vi "Actor Core.vi"(8 "error in":errorcluster, 11 "Nested in":refnum<class "UI_CAFÉ_MEX_ESP.lvclass">) -> (0 "error out":errorcluster, 3 "Actor out":refnum<class "Actor.lvclass">)   [LabVIEW 2019, in "DATA_UI_CAFÉ_MEX_ESP.lvlib" / "UI_CAFÉ_MEX_ESP.lvclass"]
doc: "(<B>Filename</B>: Actor Framework.lvlib:Actor.lvclass:Actor Core.vi)\n\nReceives messages to the actor, reacts to them, and initiates any error handling that may shut the actor down.\n\nDescendant classes may override this VI to append parallel tasks for the actor to complete while it handles messages. Overrides use the Call Parent Method node."
uses:
  C:/Program Files (x86)/National Instruments/LabVIEW 2019/vi.lib/ActorFramework/Actor/Actor.lvclass
  <vilib>/ActorFramework/Actor/Actor.lvclass
  <vilib>/ActorFramework/Actor/Actor.lvclass/Actor.ctl
  <vilib>/ActorFramework/Message Enqueuer/Message Enqueuer.lvclass/Message Enqueuer.ctl
  Write VI Refnum.vi
  <vilib>/ActorFramework/Message Enqueuer/Init from Existing Queue.vi
  <vilib>/ActorFramework/Message Enqueuer/Enqueue.vi
  <vilib>/ActorFramework/Stop Msg/Stop Msg.lvclass
  C:/Program Files (x86)/National Instruments/LabVIEW 2019/vi.lib/ActorFramework/Message/Message.lvclass
  <vilib>/ActorFramework/Message Priority Queue/Priority Enqueue.vi
  <vilib>/ActorFramework/Message Enqueuer/Message Enqueuer.lvclass
panel:
  in  "COMPRAR MERCANCÍA":bool
  in  "10 PESOS MEXICANOS":bool
  in  "5 PESOS MEXICANOS":bool
  in  "2 PESOS MEXICANOS":bool
  in  "1 PESO MEXICANO":bool
  out "CRÉDITO":dbl
  out "MONEDA":string
  out "PRODUCTO":string
  out "CANTIDAD":dbl
  out "PRECIO":dbl
  in  "SOLICITAR MERCANCIA":bool
  in  "MERCANCÍA":i32(listbox)
  # "INFORMACIÓN DEL PRODUCTO SELECCIONADO"
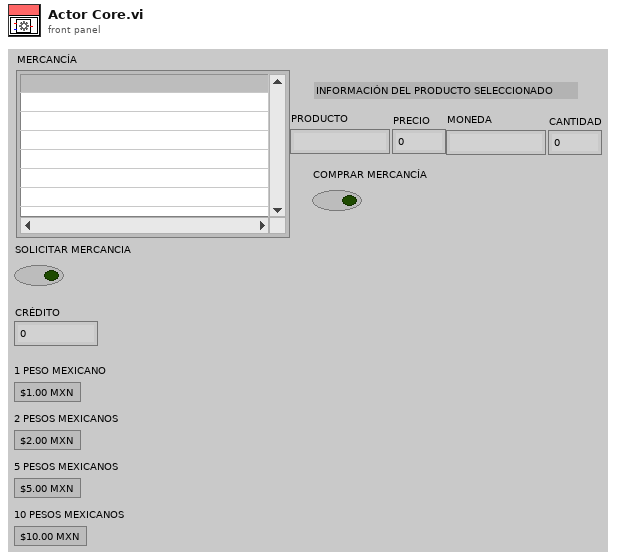
[diagram p1: front panel]
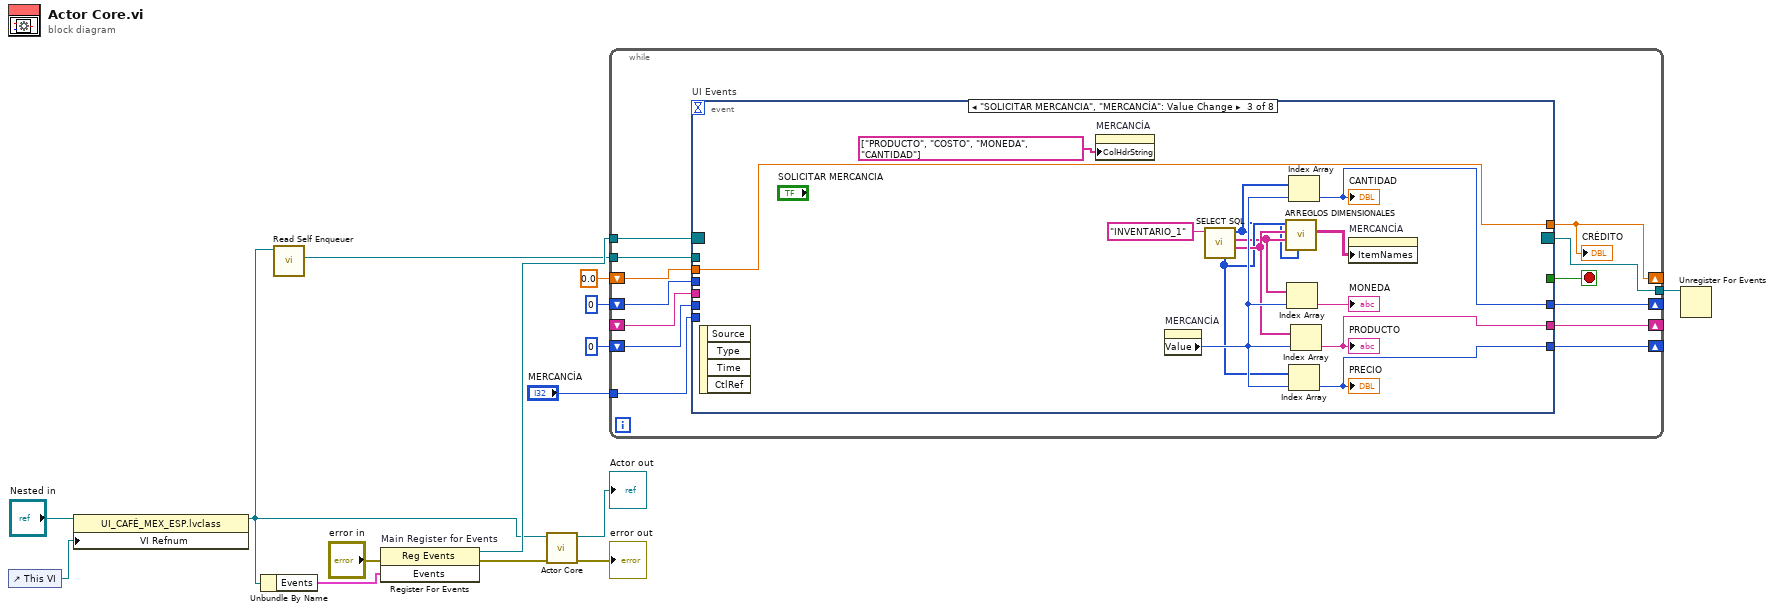
[diagram p0: block diagram]
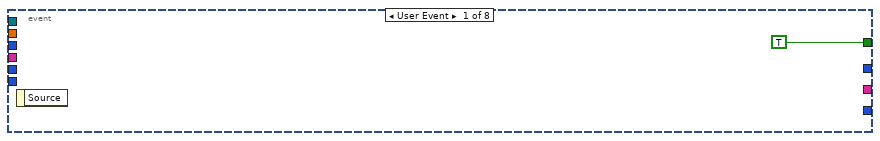
[diagram p2: hidden frame]
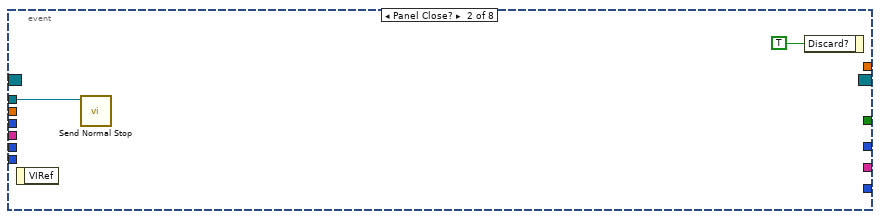
[diagram p3: hidden frame]
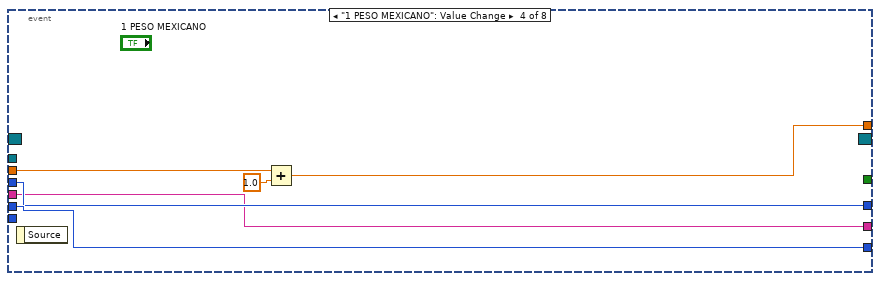
[diagram p4: hidden frame]
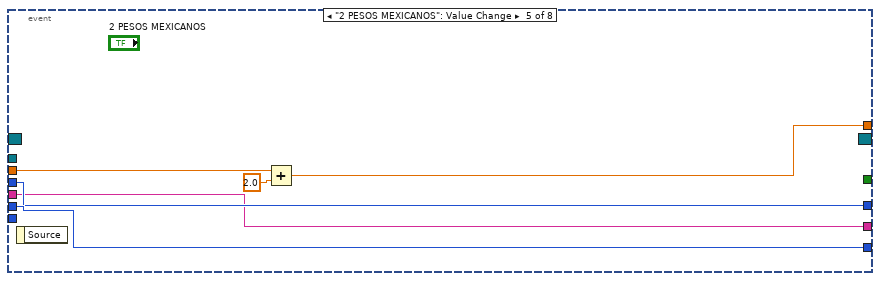
[diagram p5: hidden frame]
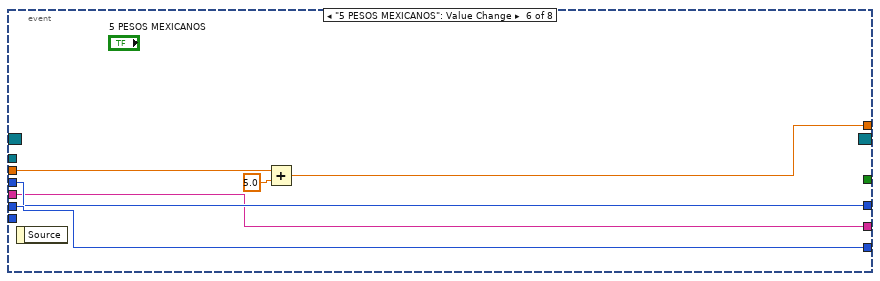
[diagram p6: hidden frame]
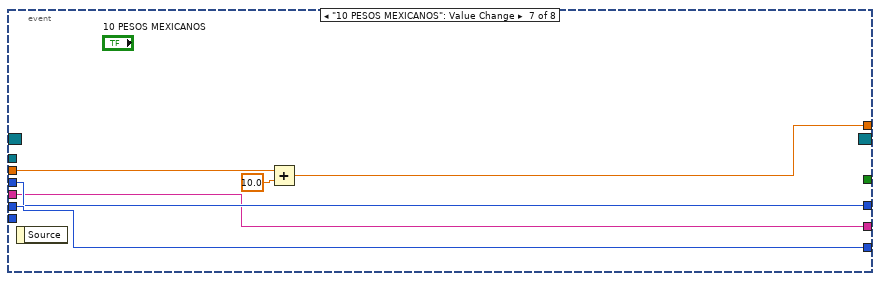
[diagram p7: hidden frame]
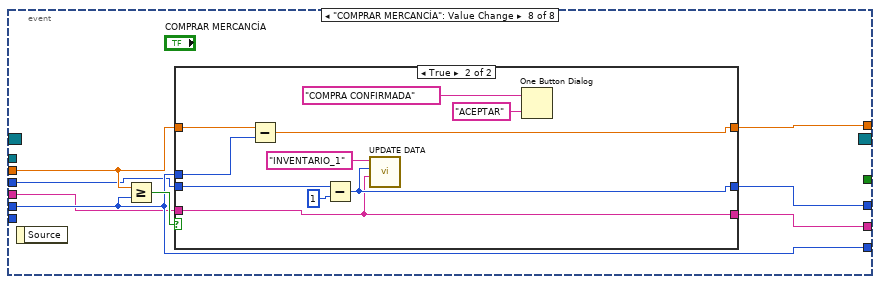
[diagram p8: hidden frame]
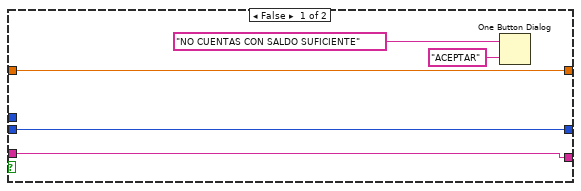
[diagram p9: hidden frame]
diagram:
  n1 = control-ref of="This VI"() -> (w5:refnum<vi>)
  n2 = property class="UI_CAFÉ_MEX_ESP.lvclass"(reference="Nested in", "VI Refnum"=w5) -> (reference out=w6:refnum<class "UI_CAFÉ_MEX_ESP.lvclass">)  [unwired: 1 in, 1 out]
  n3 = Unbundle By Name(w6) -> ("Events"=w12:cluster{"Stop":refnum<user-event>})
  n4 = call <vilib>:"Read Self Enqueuer.vi"("Actor"=w6) -> ("Self Enqueuer"=w9:refnum<class "Message Enqueuer.lvclass">)  [unwired: 10 in]
  n5 = register-events "Main Register for Events"(error in="error in", w12) -> (reference out=w13:refnum<event-registration>, error out=w7:errorcluster)  [unwired: 1 in]
  n6 = call-parent "Actor Core.vi"("error in"=w7, "Actor in"=w6) -> ("error out"=→"error out":errorcluster, "Actor out"=→"Actor out":refnum<class "Actor.lvclass">)  [unwired: 8 in]
  n7 = while {
    tunnel: w13 -> [w28]
    tunnel: [w26] -> w11
    tunnel: w9 -> [w25]
    tunnel: "MERCANCÍA" -> [w24]
    shift-right: [w22] -> _
    shift-left: 0.0 ("CRÉDITO") -> [w23]
    shift-right: [w21] -> _
    shift-left: i64 0 ("Text") -> [w20]
    shift-right: [w19] -> _
    shift-left: i64 0 ("Text") -> [w18]
    shift-right: [w17] -> _
    shift-left: _ -> [w16]
    stop <- w27 stop-if-true
    n8 = event "UI Events" shown="[2] \"SOLICITAR MERCANCIA\", \"MERCANCÍA\": Value Change" {
      selector: w28 -> [_ _ _ _ _ _ _ _]
      dyn-events: [_ _ _ _ _ _ _ _] -> w26
      timeout: _ -> [_ _ _ _ _ _ _ _]
      tunnel: [TRUE _ _ _ _ _ _ _] -> w27
      tunnel: w25 -> [_ w30 _ _ _ _ _ _]
      tunnel: w24 -> [_ _ _ _ _ _ _ _]
      tunnel: w23 -> [_ _ w32 w50 w56 w62 w68 w75]
      tunnel: [_ _ w32 w48 w54 w60 w66 w74] -> w22
      tunnel: [_ _ w35 w47 w53 w59 w65 w73] -> w21
      tunnel: w20 -> [_ _ _ w47 w53 w59 w65 w73]
      tunnel: [_ _ w34 w46 w52 w58 w64 w71] -> w19
      tunnel: w18 -> [_ _ _ w46 w52 w58 w64 w72]
      tunnel: [_ _ w33 w45 w51 w57 w63 w69] -> w17
      tunnel: w16 -> [_ _ _ w45 w51 w57 w63 w70]
      event User Event {
        n9 = event-data() -> ()  [unwired: 1 in, 1 out]
      }
      event Panel Close? {
        n10 = event-data() -> ()  [unwired: 1 in, 1 out]
        n11 = call <vilib>:"Send Normal Stop.vi"("Message Enqueuer"=w30) -> ()  [unwired: 10 in, 1 out]
        n12 = event-data("Discard?"=TRUE) -> ()  [unwired: 1 in, 1 out]
      }
      event "SOLICITAR MERCANCIA", "MERCANCÍA": Value Change {
        n13 = event-data() -> ()  [unwired: 1 in, 4 out]
        n14 = property on="MERCANCÍA" class="MCListbox (strict)"("ColHdrString"=string[] ["PRODUCTO", "COSTO", "MONEDA", "CANTIDAD"] ("Column Header Strings[]")) -> ()  [unwired: 2 in, 2 out]
        n15 = property on="MERCANCÍA" class="MCListbox (strict)"() -> ("Value"=w41:i32)  [unwired: 2 in, 2 out]
        n16 = call "SELECT SQL.vi"("INVENTARIO"="INVENTARIO_1") -> ("PRODUCTO"=w40:string[], "MONEDA"=w38:string[], "CANTIDAD"=w37:i64[], "COSTO"=w39:i64[])  [unwired: 7 in]
        n17 = call "ARREGLOS DIMENSIONALES.vi"("CANTIDAD"=w37, "MONEDA"=w38, "PRODUCTO"=w40, "COSTO"=w39) -> ("Array"=w43:string[][])  [unwired: 7 in]
        n18 = Index Array(array=w38, index=w41) -> (element=→"MONEDA":string)
        n19 = Index Array(array=w37, index=w41) -> (element=w34:i64)
        "CANTIDAD" <- w34
        n20 = Index Array(array=w39, index=w41) -> (element=w35:i64)
        "PRECIO" <- w35
        n21 = Index Array(array=w40, index=w41) -> (element=w33:string)
        "PRODUCTO" <- w33
        n22 = property on="MERCANCÍA" class="MCListbox (strict)"("ItemNames"=w43) -> ()  [unwired: 2 in, 2 out]
      }
      event "1 PESO MEXICANO": Value Change {
        n23 = event-data() -> ()  [unwired: 1 in, 1 out]
        n24 = Add(x=w50, y=1.0) -> (x+y=w48:dbl)
      }
      event "2 PESOS MEXICANOS": Value Change {
        n25 = event-data() -> ()  [unwired: 1 in, 1 out]
        n26 = Add(x=w56, y=2.0) -> (x+y=w54:dbl)
      }
      event "5 PESOS MEXICANOS": Value Change {
        n27 = event-data() -> ()  [unwired: 1 in, 1 out]
        n28 = Add(x=w62, y=5.0) -> (x+y=w60:dbl)
      }
      event "10 PESOS MEXICANOS": Value Change {
        n29 = event-data() -> ()  [unwired: 1 in, 1 out]
        n30 = Add(x=w68, y=10.0) -> (x+y=w66:dbl)
      }
      event "COMPRAR MERCANCÍA": Value Change {
        n31 = event-data() -> ()  [unwired: 1 in, 1 out]
        n32 = Greater Or Equal?(x=w75, y=w73) -> (x >= y?=w76:bool)
        n33 = case shown="True" w76 {
          tunnel: w75 -> [w79 w89]
          tunnel: w73 -> [_ w88]
          tunnel: [w79 w87] -> w74
          tunnel: w72 -> [w78 w86]
          tunnel: [w78 w83] -> w71
          tunnel: w70 -> [w77 w82]
          tunnel: [w77 w82] -> w69
          frame False {
            n34 = One Button Dialog(message="NO CUENTAS CON SALDO SUFICIENTE", button name ("OK")="ACEPTAR") -> ()  [unwired: 1 out]
          }
          frame True {
            n35 = Subtract(x=w89, y=w88) -> (x-y=w87:dbl)
            n36 = Subtract(x=w86, y=i64 1) -> (x-y=w83:i64)
            n37 = call "UPDATE DATA.vi"("PRODUCTO"=w82, "number"=w83, "TABLA"="INVENTARIO_1") -> ()  [unwired: 9 in]
            n38 = One Button Dialog(message="COMPRA CONFIRMADA", button name ("OK")="ACEPTAR") -> ()  [unwired: 1 out]
          }
        }
      }
    }
    "CRÉDITO" <- w22
  }
  n39 = Unregister For Events(event registration refnum=w11) -> ()  [unwired: 1 in, 1 out]
